vi "BMark_Create Tree.vi"(8 "error in (no error)":errorcluster, 9 "GroupByVI":bool, 10 "TreeRef":refnum<vi>, 11 "Bookmark info":T1[](array[typedef])) -> (0 "error out":errorcluster)   [LabVIEW 2016]
uses:
  <resource>/dialog/BookmarkManager/managers/Default/controls/BMark_Bookmark Data.ctl
  <resource>/dialog/BookmarkManager/managers/Default/controls/BMark_VI_Identifier.ctl
  <vilib>/addons/analyzer/_analyzerctrls.llb/VIAnCtl Analysis App Info.ctl
  <resource>/dialog/BookmarkManager/managers/Default/globals/BMark_User Visible Strings.vi
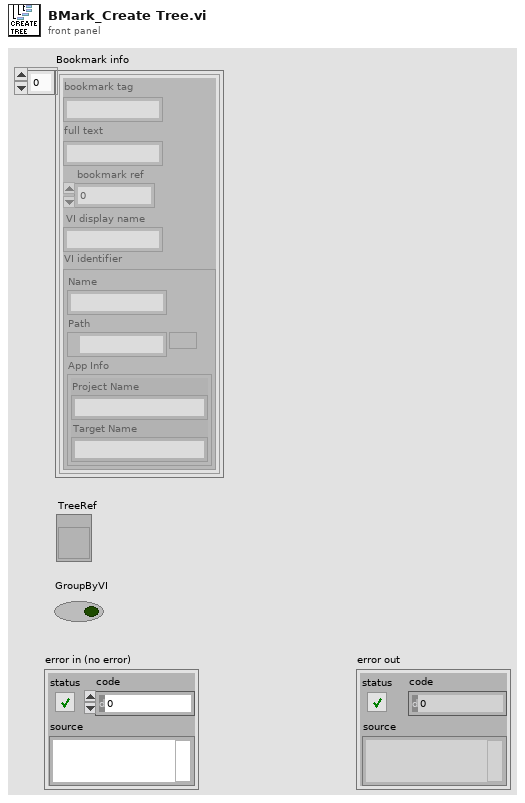
[diagram p1: front panel]
types:
  T1 = typedef "BMark_Bookmark Data.ctl" = cluster{"bookmark tag":string, "full text":string, "bookmark ref":i32, "VI display name":string, "VI identifier":T2}
  T2 = typedef "BMark_VI_Identifier.ctl" = cluster{"Name":string, "Path":path, "App Info":T3}
  T3 = typedef "VIAnCtl Analysis App Info.ctl" = cluster{"Project Name":string, "Target Name":string}
  T4 = enum8{"Enabled", "Disabled", "Disabled and Grayed Out"}
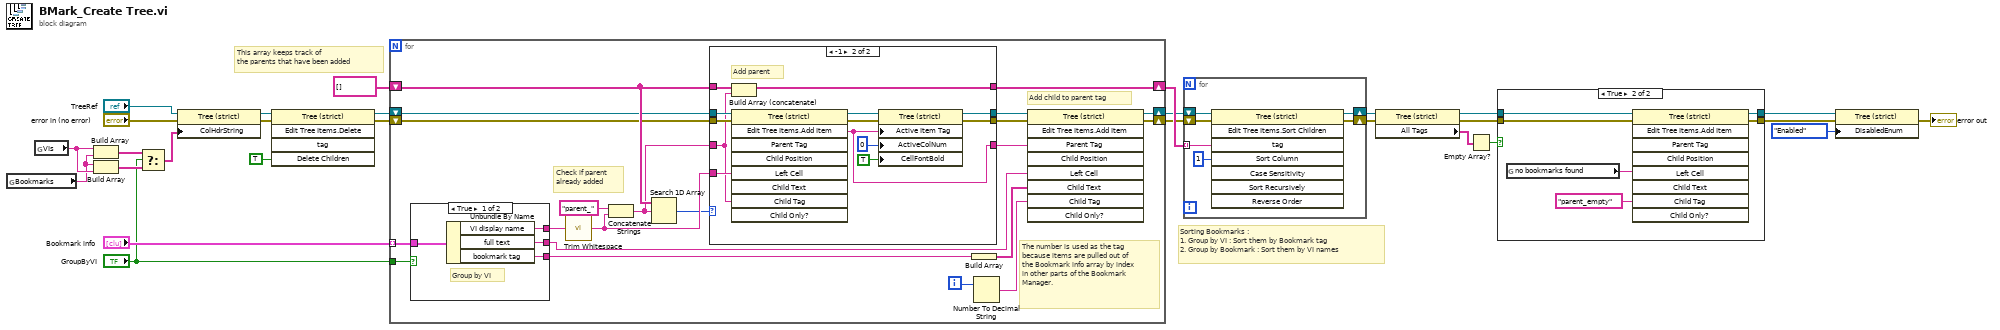
[diagram p0: block diagram]
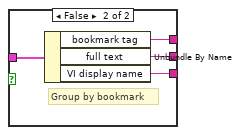
[diagram p2: hidden frame]
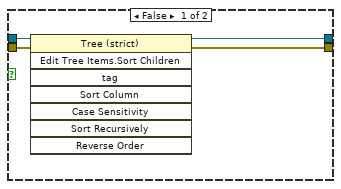
[diagram p4: hidden frame]
diagram:
  # "Sorting Bookmarks :\n1. Group by VI : Sort them by Bookmark tag\n2. Group by Bookmark : Sort them by VI names"
  # "This array keeps track of \nthe parents that have been added"
  n1 = global read "BMark_User Visible Strings.vi" "Bookmarks"() -> (w6:string)
  n2 = global read "BMark_User Visible Strings.vi" "VIs"() -> (w7:string)
  n3 = Build Array(w7, w6) -> (w19:string[])
  n4 = Build Array(w6, w7) -> (w18:string[])
  n5 = Select(t=w19, s="GroupByVI", f=w18) -> (s? t:f=w17:string[])
  n6 = property class="Tree (strict)"(reference="TreeRef", error in="error in (no error)", "ColHdrString"=w17) -> (reference out=w12:refnum<vi>, error out=w13:errorcluster)
  n7 = invoke class="Tree (strict)" method="Edit Tree Items.Delete"(reference=w12, error in=w13, "Delete Children"=TRUE ("Delete Children?")) -> (reference out=w26:refnum<vi>, error out=w27:errorcluster)  [unwired: 2 in, 3 out]
  n8 = for {
    tunnel: "Bookmark info" -> [w49] mode=indexing
    shift-right: [w47] -> w23
    shift-left: string[] [] -> [w48]
    shift-right: [w40] -> w22
    shift-left: w26 -> [w46]
    tunnel: "GroupByVI" -> [w35]
    shift-right: [w32] -> w1
    shift-left: w27 -> [w37]
    i -> [w30]
    # "The number is used as the tag because items are pulled out of the Bookmark info array by index in other parts of the Bookmark Manager."
    # "Check if parent\nalready added"
    # "Add child to parent tag"
    n9 = case shown="True" w35 {
      tunnel: w49 -> [w53 w57]
      tunnel: [w52 w56] -> w42
      tunnel: [w51 w55] -> w34
      tunnel: [w50 w54] -> w36
      frame True {
        # "Group by VI"
        n10 = Unbundle By Name(w53) -> ("VI display name"=w51:string, "full text"=w52:string, "bookmark tag"=w50:string)
      }
      frame False {
        # "Group by bookmark"
        n11 = Unbundle By Name(w57) -> ("bookmark tag"=w55:string, "full text"=w56:string, "VI display name"=w54:string)
      }
    }
    n12 = call <vilib>:"Trim Whitespace.vi"("string"=w34) -> ("trimmed string"=w33:string)  [unwired: 1 in]
    n13 = Concatenate Strings("parent_", w33) -> (w39:string)
    n14 = Search 1D Array(1D array=w48, element=w39) -> (index of element=w31:i32)  [unwired: 1 in]
    n15 = case shown="-1" w31 {
      tunnel: w48 -> [w61 w74]
      tunnel: w39 -> [w58 w67]
      tunnel: [w61 w73] -> w47
      tunnel: w37 -> [w59 w71]
      tunnel: [w59 w64] -> w38
      tunnel: w46 -> [w60 w72]
      tunnel: [w60 w63] -> w45
      tunnel: [w58 w62] -> w43
      tunnel: w33 -> [_ w70]
      frame Default {
        # "Tag previously added"
      }
      frame -1 {
        # "Add parent"
        n16 = Build Array (concatenate)(w74, w67) -> (w73:string[])
        n17 = invoke class="Tree (strict)" method="Edit Tree Items.Add Item"(reference=w72, error in=w71, "Left Cell"=w70, "Child Tag"=w67) -> (reference out=w69:refnum<vi>, error out=w68:errorcluster, "Edit Tree Items:Add Item"=w62:string)  [unwired: 5 in, 6 out]
        n18 = property class="Tree (strict)"(reference=w69, error in=w68, "Active Item Tag"=w62, "ActiveColNum"=0 ("Active Cell:Active Column Number"), "CellFontBold"=TRUE ("Active Cell:Cell Font:Bold")) -> (reference out=w63:refnum<vi>, error out=w64:errorcluster)
      }
    }
    n19 = Build Array(w36) -> (w44:string[])
    n20 = Number To Decimal String(number=w30) -> (decimal integer string=w29:string)  [unwired: 1 in]
    n21 = invoke class="Tree (strict)" method="Edit Tree Items.Add Item"(reference=w45, error in=w38, "Parent Tag"=w43, "Left Cell"=w42, "Child Text"=w44, "Child Tag"=w29) -> (reference out=w40:refnum<vi>, error out=w32:errorcluster)  [unwired: 3 in, 7 out]
  }
  n22 = for {
    tunnel: w23 -> [w79] mode=indexing
    shift-right: [w77] -> w11
    shift-left: w22 -> [w80]
    shift-right: [w78] -> w10
    shift-left: w1 -> [w76]
    n23 = invoke class="Tree (strict)" method="Edit Tree Items.Sort Children"(reference=w80, error in=w76, "tag"=w79, "Sort Column"=1) -> (reference out=w77:refnum<vi>, error out=w78:errorcluster)  [unwired: 4 in, 6 out]
  }
  n24 = property class="Tree (strict)"(reference=w11, error in=w10) -> (reference out=w21:refnum<vi>, error out=w20:errorcluster, "All Tags"=w9:string[])
  n25 = Empty Array?(array=w9) -> (empty?=w8:bool)
  n26 = case shown="True" w8 {
    tunnel: w21 -> [w84 w90]
    tunnel: w20 -> [w83 w89]
    tunnel: [w82 w88] -> w4
    tunnel: [w81 w85] -> w5
    frame False {
      n27 = invoke class="Tree (strict)" method="Edit Tree Items.Sort Children"(reference=w84, error in=w83) -> (reference out=w81:refnum<vi>, error out=w82:errorcluster)  [unwired: 6 in, 6 out]
    }
    frame True {
      n28 = global read "BMark_User Visible Strings.vi" "no bookmarks found"() -> (w86:string)
      n29 = invoke class="Tree (strict)" method="Edit Tree Items.Add Item"(reference=w90, error in=w89, "Left Cell"=w86, "Child Tag"="parent_empty") -> (reference out=w85:refnum<vi>, error out=w88:errorcluster)  [unwired: 5 in, 7 out]
    }
  }
  n30 = property class="Tree (strict)"(reference=w5, error in=w4, "DisabledEnum"=T4."Enabled" ("Disabled")) -> (error out=→"error out":errorcluster)  [unwired: 1 out]
